vi "Agilent VNA Trigger and Fetch Measurement.vi"(6 "Channel":i8=1 min=1 max=99 step=1, 7 "Agilent VNA":T1, 8 "error in (no error)":errorcluster, 10 "Timout, ms (10000)":u32=10000, 11 "VISA Resource Name":refnum<visa-resource-name>) -> (0 "error out":errorcluster, 3 "dup VISA Resource Name":refnum<visa-resource-name>)   [LabVIEW 2011]
doc: "Takes a SING sweep and returns the magnitude in dB of the requested data"
uses:
  TypeDefs/Agilent VNA Instrument Info.ctl
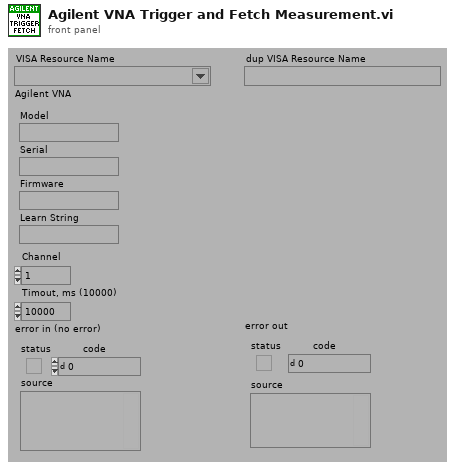
[diagram p1: front panel]
types:
  T1 = typedef "Agilent VNA Instrument Info.ctl" = cluster{"Model":string, "Serial":string, "Firmware":string, "Learn String":string}
  T2 = typedef "Agilent VNA Model.ctl" = enum16{"Not Supported", "8510X", "8719X", "8720X", "8722X", "8753X", "ENA", "PNA", "Field Fox"}
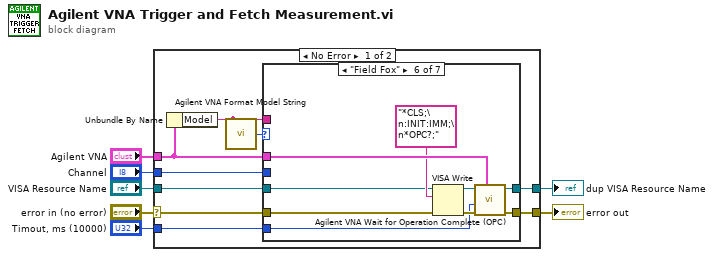
[diagram p0: block diagram]
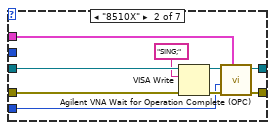
[diagram p3: hidden frame]
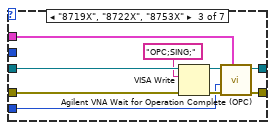
[diagram p4: hidden frame]
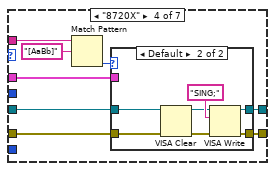
[diagram p5: hidden frame]
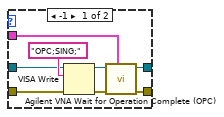
[diagram p6: hidden frame]
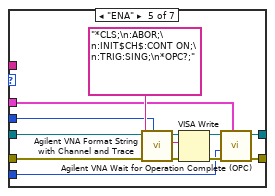
[diagram p7: hidden frame]
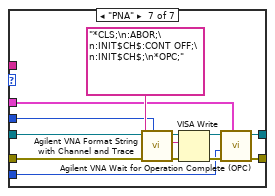
[diagram p8: hidden frame]
diagram:
  n1 = case shown="No Error" "error in (no error)" {
    selector: "error in (no error)" -> [w15 w92]
    tunnel: "VISA Resource Name" -> [w16 w91]
    tunnel: "Timout, ms (10000)" -> [w14 _]
    tunnel: [w13 w92] -> w4
    tunnel: [w12 w91] -> w5
    tunnel: "Agilent VNA" -> [w9 _]
    tunnel: "Channel" -> [w10 _]
    frame No Error {
      n2 = Unbundle By Name(w9) -> ("Model"=w8:string)
      n3 = call "Agilent VNA Format Model String.vi"("Model"=w8) -> ("Model"=w11:T2)
      n4 = case shown="\"Field Fox\"" w11 {
        tunnel: w16 -> [w18 w27 w36 w41 w70 w71 w90]
        tunnel: w15 -> [w17 w25 w34 w42 w69 w79 w89]
        tunnel: w14 -> [_ w22 w31 _ w61 w72 w81]
        tunnel: [w17 w21 w30 w44 w63 w75 w83] -> w13
        tunnel: [w18 w20 w29 w43 w64 w76 w84] -> w12
        tunnel: w10 -> [_ _ _ _ w60 _ w80]
        tunnel: w9 -> [_ w19 w28 w37 w62 w74 w82]
        tunnel: w8 -> [_ _ _ w39 _ _ _]
        frame "Not Supported" {
        }
        frame "8510X" {
          n5 = VISA Write(VISA resource name=w27, write buffer="SING;" ("write buffer (\"\")"), error in (no error)=w25) -> (VISA resource name out=w24:refnum<visa-resource-name>, error out=w23:errorcluster)  [unwired: 1 out]
          n6 = call "Agilent VNA Wait for Operation Complete (OPC).vi"("Agilent VNA"=w19, "error in (no error)"=w23, "Timeout, ms (10000)"=w22, "VISA Resource Name"=w24) -> ("error out"=w21:errorcluster, "dup VISA Resource Name"=w20:refnum<visa-resource-name>)  [unwired: 6 out]
        }
        frame "8719X", "8722X", "8753X" {
          n7 = VISA Write(VISA resource name=w36, write buffer="OPC;SING;" ("write buffer (\"\")"), error in (no error)=w34) -> (VISA resource name out=w33:refnum<visa-resource-name>, error out=w32:errorcluster)  [unwired: 1 out]
          n8 = call "Agilent VNA Wait for Operation Complete (OPC).vi"("Agilent VNA"=w28, "error in (no error)"=w32, "Timeout, ms (10000)"=w31, "VISA Resource Name"=w33) -> ("error out"=w30:errorcluster, "dup VISA Resource Name"=w29:refnum<visa-resource-name>)  [unwired: 6 out]
        }
        frame "8720X" {
          n9 = Match Pattern(string=w39, regular expression="[AaBb]") -> (offset past match=w38:i32)  [unwired: 4 out]
          n10 = case shown="Default" w38 {
            tunnel: [w47 w59] -> w44
            tunnel: [w46 w58] -> w43
            tunnel: w42 -> [w48 w56]
            tunnel: w41 -> [w49 w55]
            tunnel: w37 -> [w45 _]
            frame -1 {
              n11 = VISA Write(VISA resource name=w49, write buffer="OPC;SING;" ("write buffer (\"\")"), error in (no error)=w48) -> (VISA resource name out=w51:refnum<visa-resource-name>, error out=w50:errorcluster)  [unwired: 1 out]
              n12 = call "Agilent VNA Wait for Operation Complete (OPC).vi"("Agilent VNA"=w45, "error in (no error)"=w50, "VISA Resource Name"=w51) -> ("error out"=w47:errorcluster, "dup VISA Resource Name"=w46:refnum<visa-resource-name>)  [unwired: 1 in, 6 out]
            }
            frame Default {
              n13 = VISA Clear(VISA resource name=w55, error in (no error)=w56) -> (VISA resource name out=w54:refnum<visa-resource-name>, error out=w53:errorcluster)
              n14 = VISA Write(VISA resource name=w54, write buffer="SING;", error in (no error)=w53) -> (VISA resource name out=w58:refnum<visa-resource-name>, error out=w59:errorcluster)  [unwired: 1 out]
            }
          }
        }
        frame "ENA" {
          n15 = call "Agilent VNA Format String with Channel and Trace.vi"("Channel"=w60, "String"="*CLS;\n:ABOR;\n:INIT$CH$:CONT ON;\n:TRIG:SING;\n*OPC?;" ("write buffer")) -> ("String Out"=w67:string)  [unwired: 1 in, 6 out]
          n16 = VISA Write(VISA resource name=w70, write buffer=w67, error in (no error)=w69) -> (VISA resource name out=w65:refnum<visa-resource-name>, error out=w66:errorcluster)  [unwired: 1 out]
          n17 = call "Agilent VNA Wait for Operation Complete (OPC).vi"("Agilent VNA"=w62, "error in (no error)"=w66, "Timeout, ms (10000)"=w61, "VISA Resource Name"=w65) -> ("error out"=w63:errorcluster, "dup VISA Resource Name"=w64:refnum<visa-resource-name>)  [unwired: 6 out]
        }
        frame "Field Fox" {
          n18 = VISA Write(VISA resource name=w71, write buffer="*CLS;\n:INIT:IMM;\n*OPC?;", error in (no error)=w79) -> (VISA resource name out=w77:refnum<visa-resource-name>, error out=w78:errorcluster)  [unwired: 1 out]
          n19 = call "Agilent VNA Wait for Operation Complete (OPC).vi"("Agilent VNA"=w74, "error in (no error)"=w78, "Timeout, ms (10000)"=w72, "VISA Resource Name"=w77) -> ("error out"=w75:errorcluster, "dup VISA Resource Name"=w76:refnum<visa-resource-name>)  [unwired: 6 out]
        }
        frame "PNA" {
          n20 = call "Agilent VNA Format String with Channel and Trace.vi"("Channel"=w80, "String"="*CLS;\n:ABOR;\n:INIT$CH$:CONT OFF;\n:INIT$CH$;\n*OPC;" ("write buffer")) -> ("String Out"=w87:string)  [unwired: 1 in, 6 out]
          n21 = VISA Write(VISA resource name=w90, write buffer=w87, error in (no error)=w89) -> (VISA resource name out=w85:refnum<visa-resource-name>, error out=w86:errorcluster)  [unwired: 1 out]
          n22 = call "Agilent VNA Wait for Operation Complete (OPC).vi"("Agilent VNA"=w82, "error in (no error)"=w86, "Timeout, ms (10000)"=w81, "VISA Resource Name"=w85) -> ("error out"=w83:errorcluster, "dup VISA Resource Name"=w84:refnum<visa-resource-name>)  [unwired: 6 out]
        }
      }
    }
    frame Error {
      # "Incoming Error....do nothing."
    }
  }
  "dup VISA Resource Name" <- w5
  "error out" <- w4
